vi "GripperStringFormat.vi"(10 "String IN":string) -> (2 "String OUT":string)   [LabVIEW 2020]
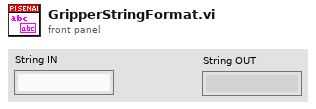
[diagram p1: front panel]
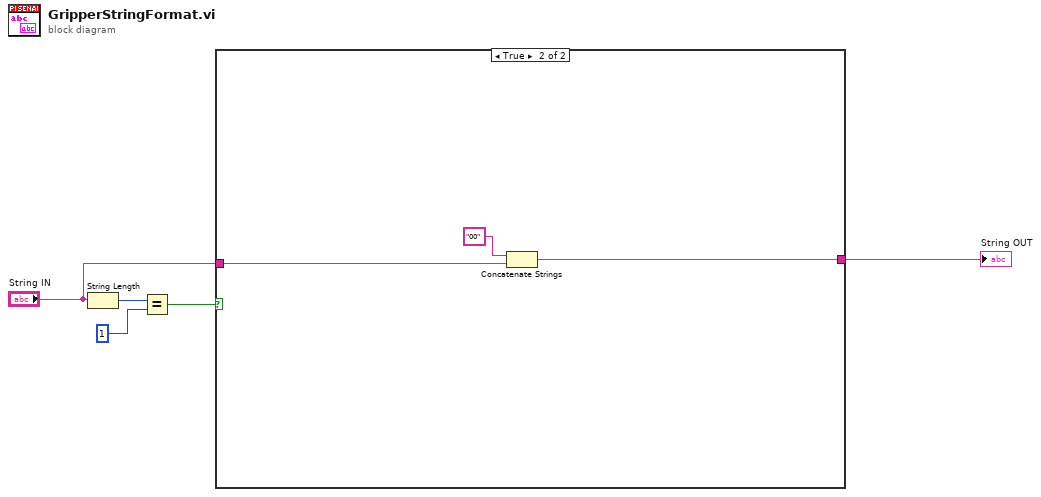
[diagram p0: block diagram]
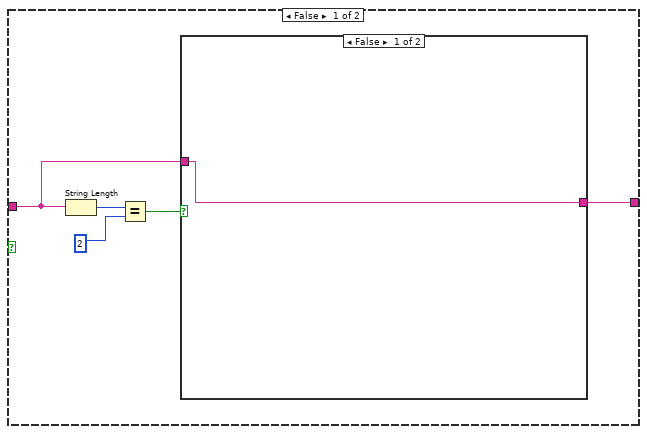
[diagram p2: hidden frame]
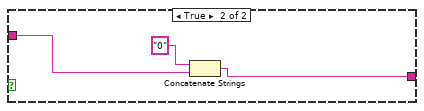
[diagram p3: hidden frame]
diagram:
  n1 = String Length(string="String IN") -> (length=w5:i32)
  n2 = Equal?(x=w5, y=1) -> (x = y?=w3:bool)
  n3 = case shown="True" w3 {
    tunnel: "String IN" -> [w6 w16]
    tunnel: [w7 w15] -> w1
    frame False {
      n4 = String Length(string=w6) -> (length=w9:i32)
      n5 = Equal?(x=w9, y=2) -> (x = y?=w8:bool)
      n6 = case shown="False" w8 {
        tunnel: [w11 w13] -> w7
        tunnel: w6 -> [w11 w12]
        frame False {
        }
        frame True {
          n7 = Concatenate Strings("0" ("string"), w12) -> (w13:string)
        }
      }
    }
    frame True {
      n8 = Concatenate Strings("00" ("string"), w16) -> (w15:string)
    }
  }
  "String OUT" <- w1
